vi "Poll.vi"() -> ()   [LabVIEW 2014]
uses:
  <vilib>/addons/zeromq/poll_type.ctl
  <vilib>/addons/zeromq/socket_type.ctl
  <vilib>/addons/zeromq/socket_options.ctl
  <userlib>/_OpenG.lib/numeric/numeric.llb/Random Number Within Range - DBL__ogtk.vi
  <vilib>/addons/zeromq/zmq_poll_scalar.vi
  <vilib>/addons/zeromq/zmq_context.lvclass
  <vilib>/addons/zeromq/zeromq.lvlib
  <vilib>/addons/zeromq/zmq_socket.lvclass
panel:
  out "data":string
  in  "stop":bool
  out "timed out?":bool
  out "nevents":i32
  out "current time":timestamp
  out "polled events":T1[](array[typedef])
  out "string":string
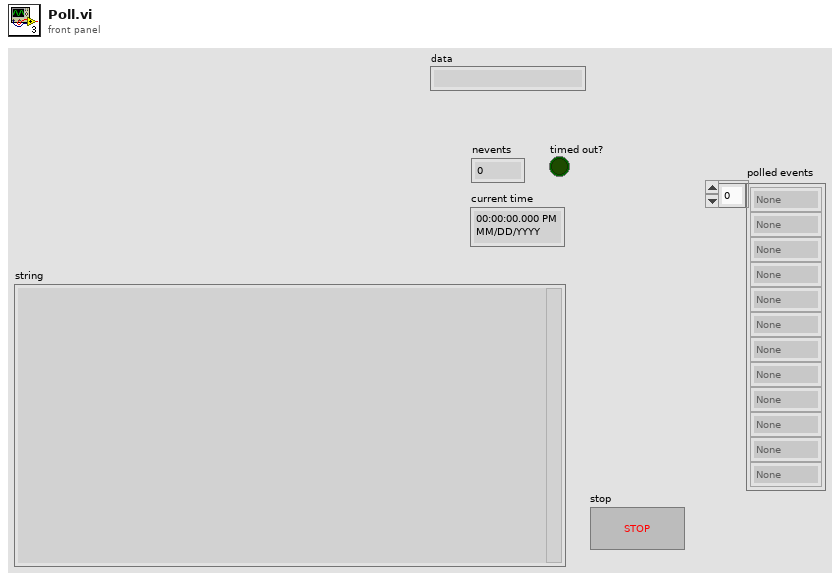
[diagram p1: front panel]
types:
  T1 = typedef "zeromq.lvlib/poll_type.ctl" = enum16{"None", "In", "Out", "In/Out"}
  T2 = typedef "zeromq.lvlib/socket_options.ctl" = enum8{"NONE", "ZMQ_HWM", "<2>", "ZMQ_SWAP", "ZMQ_AFFINITY", "ZMQ_IDENTITY", "ZMQ_SUBSCRIBE", "ZMQ_UNSUBSCRIBE", "ZMQ_RATE", "ZMQ_RECOVERY_IVL", "ZMQ_MCAST_LOOP", "ZMQ_SNDBUF", "ZMQ_RCVBUF", "ZMQ_RCVMORE", "ZMQ_FD", "ZMQ_EVENTS", "ZMQ_TYPE", "ZMQ_LINGER", "ZMQ_RECONNECT_IVL", "ZMQ_BACKLOG", "ZMQ_RECOVERY_IVL_MSEC", "ZMQ_RECONNECT_IVL_MAX", "ZMQ_MAXMSGSIZE", "ZMQ_SNDHWM", "ZMQ_RCVHWM", "ZMQ_MULTICAST_HOPS", "<26>", "ZMQ_RCVTIMEO", "ZMQ_SNDTIMEO", "<29>", "<30>", "ZMQ_IPV4ONLY", "ZMQ_LAST_ENDPOINT", "ZMQ_ROUTER_MANDATORY", "ZMQ_TCP_KEEPALIVE", "ZMQ_TCP_KEEPALIVE_CNT", "ZMQ_TCP_KEEPALIVE_IDLE", "ZMQ_TCP_KEEPALIVE_INTVL", "ZMQ_TCP_ACCEPT_FILTER", "ZMQ_DELAY_ATTACH_ON_CONNECT", "ZMQ_XPUB_VERBOSE"}
  T3 = typedef "zeromq.lvlib/socket_type.ctl" = enum8{"ZMQ_PAIR", "ZMQ_PUB", "ZMQ_SUB", "ZMQ_REQ", "ZMQ_REP", "ZMQ_DEALER", "ZMQ_ROUTER", "ZMQ_PULL", "ZMQ_PUSH", "ZMQ_XPUB", "ZMQ_XSUB"}
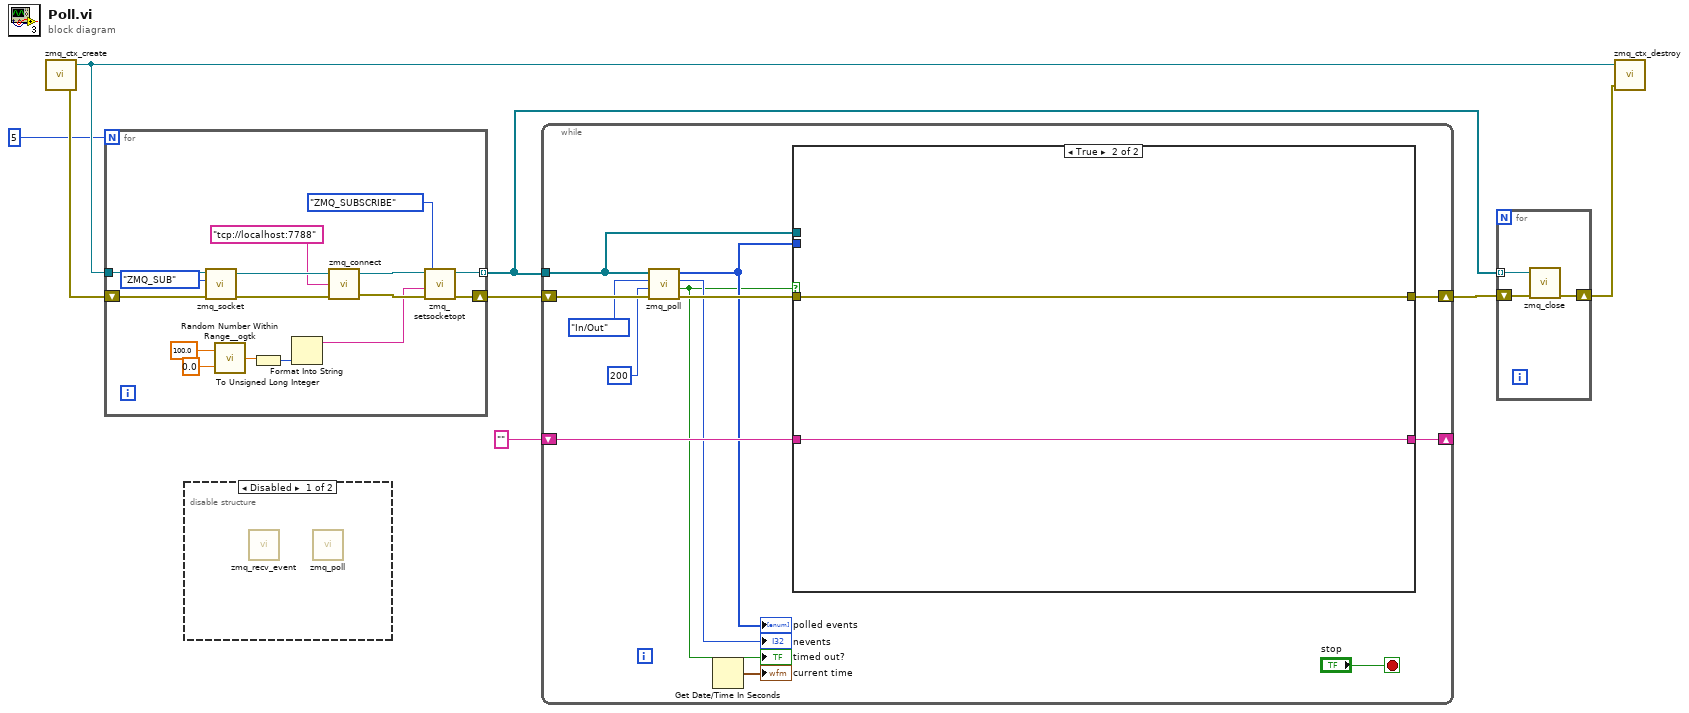
[diagram p0: block diagram]
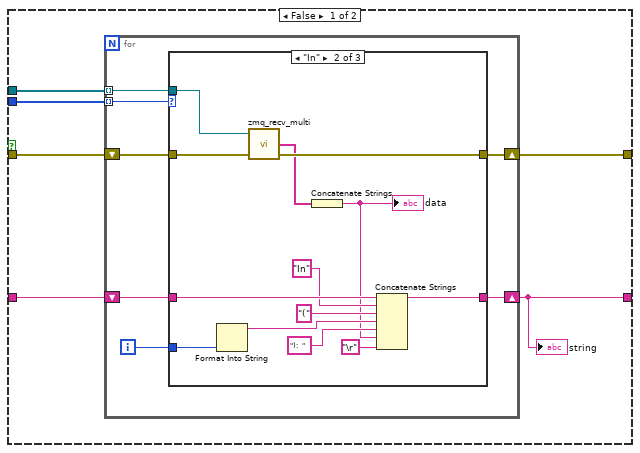
[diagram p3: hidden frame]
diagram:
  n1 = call <vilib>:"zmq_ctx_create.vi"() -> ("error out"=w8:errorcluster, "context out"=w7:refnum<class "zmq_context.lvclass">)  [unwired: 4 in]
  n2 = for {
    N: 5 -> [_]
    tunnel: w7 -> [w22]
    tunnel: [w17] -> w3 mode=indexing
    shift-right: [w15] -> w2
    shift-left: w8 -> [w23]
    n3 = call <vilib>:"zmq_socket.vi"("error in"=w23, "socket type"=socket_type."ZMQ_SUB", "context in"=w22) -> ("error out"=w20:errorcluster, "socket out"=w21:refnum<class "zmq_socket.lvclass">)  [unwired: 2 in, 1 out]
    n4 = call-poly <userlib>:"Random Number Within Range__ogtk.vi"("High"=100.0, "Low"=0.0) -> ("Random Number"=w11:dbl)  [unwired: 3 in]
    n5 = To Unsigned Long Integer(number=w11) -> (unsigned 32bit integer=w10:u32)
    n6 = Format Into String(w10) -> (resulting string=w9:string)  [unwired: 3 in, 1 out]
    n7 = call <vilib>:"zmq_connect.vi"("error in"=w20, "endpoint"="tcp://localhost:7788", "socket in"=w21) -> ("error out"=w16:errorcluster, "socket out"=w18:refnum<class "zmq_socket.lvclass">)  [unwired: 1 in]
    n8 = call <vilib>:"zmq_setsocketopt.vi"("error in"=w16, "value"=w9, "option"=socket_options."ZMQ_SUBSCRIBE", "socket in"=w18) -> ("error out"=w15:errorcluster, "socket out"=w17:refnum<class "zmq_socket.lvclass">)  [unwired: 2 in]
  }
  n9 = disable-structure shown="Disabled" {
    frame Disabled {
      n10 = call <vilib>:"zmq_recv_event.vi"() -> ()  [unwired: 6 in, 2 out]
      n11 = call-poly <vilib>:"zmq_poll.vi"() -> ()  [unwired: 4 in, 4 out]
    }
    frame Enabled {
    }
  }
  n12 = while {
    shift-right: [w37] -> w6
    shift-left: w2 -> [w34]
    shift-right: [w35] -> _
    shift-left: "" -> [w36]
    tunnel: w3 -> [w27]
    stop <- "stop" stop-if-true
    n13 = call-poly <vilib>:"zmq_poll.vi"("error in"=w34, "timeout"=200, "poll type"=poll_type."In/Out", "sockets"=w27) -> ("error out"=w33:errorcluster, "timed out?"=w25:bool, "nevents"=→"nevents":i32, "polled events"=w32:T1[])
    "polled events" <- w32
    "timed out?" <- w25
    n14 = Get Date/Time In Seconds() -> (seconds since 1Jan1904=→"current time":timestamp)
    n15 = case shown="True" w25 {
      tunnel: [w43 w68] -> w37
      tunnel: w36 -> [w42 w69]
      tunnel: [w41 w69] -> w35
      tunnel: w33 -> [w40 w68]
      tunnel: w32 -> [w39 _]
      tunnel: w27 -> [w38 _]
      frame False {
        n16 = for {
          tunnel: w38 -> [w47] mode=indexing
          tunnel: w39 -> [w50] mode=indexing
          shift-right: [w49] -> w43
          shift-left: w40 -> [w48]
          shift-right: [w46] -> w41
          shift-left: w42 -> [w45]
          i -> [w44]
          n17 = case shown="\"In\"" w50 {
            tunnel: [w52 w63 w67] -> w49
            tunnel: w48 -> [w52 w65 w67]
            tunnel: w47 -> [_ w64 _]
            tunnel: [w51 w61 w66] -> w46
            tunnel: w45 -> [w51 w62 w66]
            tunnel: w44 -> [_ w57 _]
            frame "None", Default {
            }
            frame "In" {
              n18 = Format Into String(w57) -> (resulting string=w56:string)  [unwired: 3 in, 1 out]
              n19 = call <vilib>:"zmq_recv_multi.vi"("error in"=w65, "socket in"=w64) -> ("error out"=w63:errorcluster, "parts"=w55:string[])  [unwired: 1 in, 1 out]
              n20 = Concatenate Strings(w55) -> (w53:string)
              "data" <- w53
              n21 = Concatenate Strings(w62, "In" ("string"), "(" ("string"), w56, "):  " ("string"), w53, "\r") -> (w61:string)
            }
            frame "Out" {
            }
          }
        }
        "string" <- w41
      }
      frame True {
      }
    }
  }
  n22 = for {
    tunnel: w3 -> [w70] mode=indexing
    shift-right: [w71] -> w5
    shift-left: w6 -> [w72]
    n23 = call <vilib>:"zmq_close.vi"("error in"=w72, "socket"=w70) -> ("error out"=w71:errorcluster)  [unwired: 3 in]
  }
  n24 = call <vilib>:"zmq_ctx_destroy.vi"("error in"=w5, "context in"=w7) -> ()  [unwired: 3 in, 1 out]
